vi "initialise.vi"(8 "error in (no error)":errorcluster, 11 "DL090216Display in":refnum<class "DisplayDL090216.lvclass">) -> (0 "error out":errorcluster, 3 "DL090216Display out":refnum<class "DisplayDL090216.lvclass">)   [LabVIEW 2010, in "DisplayDL090216.lvclass"]
uses:
  DisplayDL090216.lvclass
  common/enumerations/top-level_component_type_enum.ctl
  GenericDisplay/GenericDisplay/GenericDisplay.lvclass
  ImageProcessor/GenericImageProcessor/GenericImageProcessor/GenericImageProcessor.lvclass
  Command/GenericImageProcessorChangedCommand/GenericImageProcessorChangedCommand/GenericImageProcessorChangedCommand.lvclass
  UpdateDisplayDL090216Command/UpdateDisplayDL090216Command.lvclass
  common/classes/Image/Image/Image.lvclass
  DisplayDL090216.lvclass/DisplayDL090216.ctl
  common/classes/ColorOverlay/ColorOverlay/ColorOverlay.lvclass
  common/classes/ErrorController/ErrorController/class_data.vi
  common/classes/ErrorController/ErrorController/ErrorController.lvclass
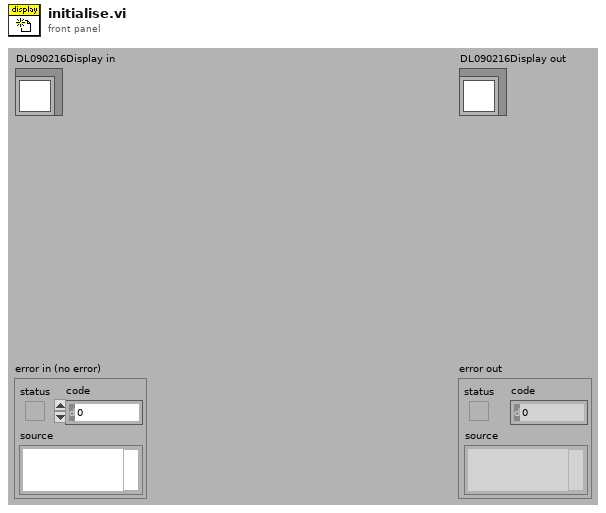
[diagram p1: front panel]
types:
  T1 = typedef "top-level_component_type_enum.ctl" = enum16{"undefined", "ImagingMode", "ScanHead", "DAQ", "ImageAssembler", "Display", "DataCollection", "Analyser", "Stimulator", "ExperimentController", "Instrument", "Stage"}
  T2 = typedef "Image Type" = u32
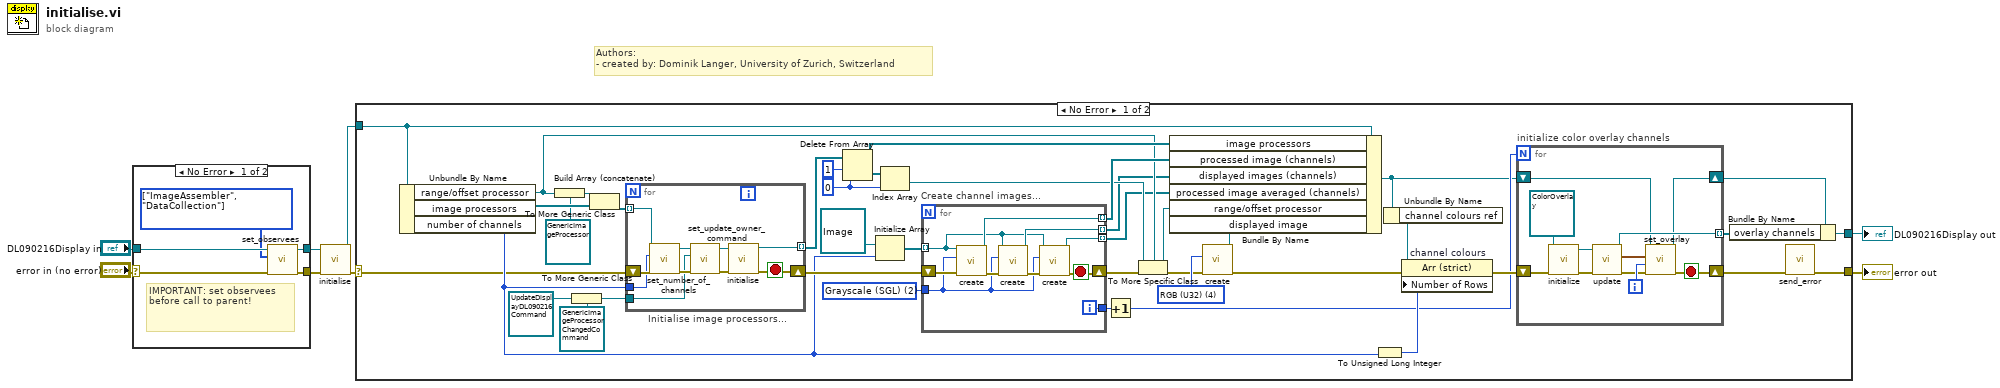
[diagram p0: block diagram]
diagram:
  # "Authors: \n- created by: Dominik Langer, University of Zurich, Switzerland"
  n1 = case shown="No Error" "error in (no error)" {
    selector: "error in (no error)" -> [w10 w14]
    tunnel: "DL090216Display in" -> [w13 w15]
    tunnel: [w12 w15] -> w3
    tunnel: [w11 w14] -> w2
    frame No Error {
      w9 = T1[] [enum."ImageAssembler", enum."DataCollection"] items=["undefined", "ImagingMode", "ScanHead", "DAQ", "ImageAssembler", "Display", "DataCollection", "Analyser", "Stimulator", "ExperimentController", "Instrument", "Stage"] ("observees")
      # "IMPORTANT: set observees before call to parent!"
      n2 = call-dynamic "set_observees.vi"("error in (no error)"=w10, "observees"=w9, "GenericToplevelComponent in"=w13) -> ("error out"=w11:errorcluster, "GenericToplevelComponent out"=w12:refnum<class "DisplayDL090216.lvclass">)  [unwired: 7 in]
    }
    frame Error {
    }
  }
  n3 = call-parent "initialise.vi"("error in (no error)"=w2, "GenericPlugin in"=w3) -> ("error out"=w6:errorcluster, "GenericPlugin out"=w5:refnum<class "DisplayDL090216.lvclass">)  [unwired: 8 out]
  n4 = case shown="No Error" w6 {
    selector: w6 -> [w18 w89]
    tunnel: [w25 w89] -> w8
    tunnel: [w30 w88] -> w7
    tunnel: w5 -> [w17 w88]
    frame No Error {
      w47 = 0 ("index")
      w54 = T2 4 items=["Grayscale (U8)", "Grayscale (I16)", "Grayscale (SGL)", "Complex (CSG)", "RGB (U32)", "HSL (U32)", "RGB (U64)", "Grayscale (U16)"] ("Image Type")
      w55 = T2 2 items=["Grayscale (U8)", "Grayscale (I16)", "Grayscale (SGL)", "Complex (CSG)", "RGB (U32)", "HSL (U32)", "RGB (U64)", "Grayscale (U16)"] ("Image Type")
      n5 = Unbundle By Name(w17) -> ("range/offset processor"=w38:refnum<class "ImageProcessorDL090216RangeOffset.lvclass">, "image processors"=w40:refnum<class "GenericImageProcessor.lvclass">[], "number of channels"=w20:i32)
      n6 = To More Generic Class(target class=refnum<class "GenericImageProcessor.lvclass"> refnum ("GenericImageProcessor.lvclass"), reference=w38) -> (generic class reference=w37:refnum<class "GenericImageProcessor.lvclass">)
      n7 = To More Generic Class(target class=refnum<class "GenericImageProcessorChangedCommand.lvclass"> refnum ("GenericImageProcessorChangedCommand.lvclass"), reference=refnum<class "UpdateDisplayDL090216Command.lvclass"> refnum ("UpdateDL090216DisplayCommand.lvclass")) -> (generic class reference=w51:refnum<class "GenericImageProcessorChangedCommand.lvclass">)
      n8 = Build Array (concatenate)(w37, w40) -> (w39:refnum<class "GenericImageProcessor.lvclass">[])
      n9 = for "Initialise image processors..." {
        shift-right: [w69] -> w22
        shift-left: w18 -> [w77]
        tunnel: w39 -> [w76] mode=indexing
        tunnel: [w70] -> w49 mode=indexing
        tunnel: w51 -> [w71]
        tunnel: w20 -> [w68]
        stop <- w69 stop-if-true
        n10 = call "set_number_of_channels.vi"("error in (no error)"=w77, "number of channels"=w68, "GenericImageProcessor.lvclass in"=w76) -> ("error out"=w75:errorcluster, "GenericImageProcessor.lvclass out"=w74:refnum<class "GenericImageProcessor.lvclass">)  [unwired: 7 out]
        n11 = call-dynamic "set_update_owner_command.vi"("error in (no error)"=w75, "update-owner command"=w71, "GenericImageProcessor.lvclass in"=w74) -> ("error out"=w73:errorcluster, "GenericImageProcessor.lvclass out"=w72:refnum<class "GenericImageProcessor.lvclass">)  [unwired: 7 out]
        n12 = call-dynamic "initialise.vi"("error in (no error)"=w73, "GenericImageProcessor in"=w72) -> ("error out"=w69:errorcluster, "GenericImageProcessor out"=w70:refnum<class "GenericImageProcessor.lvclass">)  [unwired: 8 out]
      }
      n13 = Delete From Array(array=w49, length=1, index=w47) -> (deleted portion=w46:refnum<class "GenericImageProcessor.lvclass">[], array with subset deleted=w45:refnum<class "GenericImageProcessor.lvclass">[])
      n14 = Initialize Array(refnum<class "Image.lvclass"> refnum ("Image.lvclass"), w20) -> (w35:refnum<class "Image.lvclass">[])
      n15 = Index Array(array=w46, index=w47) -> (element=w42:refnum<class "GenericImageProcessor.lvclass">)
      n16 = for "Create channel images..." {
        shift-right: [w81] -> w44
        shift-left: w22 -> [w87]
        tunnel: w35 -> [w79] mode=indexing
        tunnel: w55 -> [w80]
        tunnel: [w86] -> w53 mode=indexing
        tunnel: [w84] -> w34 mode=indexing
        tunnel: [w83] -> w24
        tunnel: [w78] -> w16 mode=indexing
        i -> [w83]
        stop <- w81 stop-if-true
        n17 = call "create.vi"("error in (no error)"=w87, "Image Type"=w80, "Image in"=w79) -> ("error out"=w85:errorcluster, "Image out"=w86:refnum<class "Image.lvclass">)  [unwired: 1 in, 6 out]
        n18 = call "create.vi"("error in (no error)"=w85, "Image Type"=w80, "Image in"=w79) -> ("error out"=w82:errorcluster, "Image out"=w84:refnum<class "Image.lvclass">)  [unwired: 1 in, 6 out]
        n19 = call "create.vi"("error in (no error)"=w82, "Image Type"=w80, "Image in"=w79) -> ("error out"=w81:errorcluster, "Image out"=w78:refnum<class "Image.lvclass">)  [unwired: 1 in, 6 out]
      }
      n20 = Increment(x=w24) -> (x+1=w23:i32)
      n21 = To More Specific Class(target class=w38, reference=w42, error in=w44) -> (specific class reference=w41:refnum<class "ImageProcessorDL090216RangeOffset.lvclass">, error out=w43:errorcluster)
      n22 = call "create.vi"("error in (no error)"=w43, "Image Type"=w54) -> ("error out"=w21:errorcluster, "Image out"=w33:refnum<class "Image.lvclass">)  [unwired: 2 in, 6 out]
      n23 = Bundle By Name(cluster=w17, "image processors"=w45, "processed image (channels)"=w53, "displayed images (channels)"=w34, "processed image averaged (channels)"=w16, "range/offset processor"=w41, "displayed image"=w33) -> (w19:refnum<class "DisplayDL090216.lvclass">)
      n24 = To Unsigned Long Integer(number=w20) -> (unsigned 32bit integer=w31:u32)
      n25 = Unbundle By Name(w19) -> ("channel colours ref"=w32:refnum<vi>)
      n26 = property on="channel colours" class="Arr (strict)"(reference=w32, error in=w21, "Number of Rows"=w31) -> (error out=w28:errorcluster)  [unwired: 1 out]
      n27 = for "initialize color overlay channels" {
        N: w23 -> [_]
        shift-right: [w61] -> w26
        shift-left: w28 -> [w59]
        tunnel: [w66] -> w29 mode=indexing
        shift-right: [w63] -> w27
        shift-left: w19 -> [w64]
        i -> [w67]
        stop <- w61 stop-if-true
        n28 = call-dynamic "initialize.vi"("error in (no error)"=w59, "ColorOverlay in"=refnum<class "ColorOverlay.lvclass"> refnum ("ColorOverlay.lvclass")) -> ("error out"=w58:errorcluster, "ColorOverlay out"=w57:refnum<class "ColorOverlay.lvclass">)  [unwired: 8 in]
        n29 = call-dynamic "update.vi"("error in (no error)"=w58, "ColorOverlay in"=w57) -> ("error out"=w62:errorcluster, "color cluster out"=w65:cluster{"Red":u8, "Green":u8, "Blue":u8}[], "ColorOverlay out"=w66:refnum<class "ColorOverlay.lvclass">)  [unwired: 7 in]
        n30 = call-dynamic "set_overlay.vi"("error in (no error)"=w62, "raw channel index"=w67, "palette in"=w65, "DisplayDL090216 in"=w64) -> ("error out"=w61:errorcluster, "DisplayDL090216 out"=w63:refnum<class "DisplayDL090216.lvclass">)  [unwired: 6 in]
      }
      n31 = Bundle By Name(cluster=w27, "overlay channels"=w29) -> (w30:refnum<class "DisplayDL090216.lvclass">)
      n32 = call "send_error.vi"("error in (no error)"=w26) -> ("error out"=w25:errorcluster)  [unwired: 10 in]
    }
    frame Error {
    }
  }
  "error out" <- w8
  "DL090216Display out" <- w7
